vi "OP300ZP_CONTI_HYDRAU.vi"(6 "last?":bool, 7 "OUI/NON":bool, 8 "errin":errorcluster caption="entrée d'erreur (pas d'erreur)", 11 "cluster d'entrée":T1) -> (0 "errout":errorcluster caption="sortie d'erreur")   [LabVIEW 2020]
uses:
  <userlib>/Alex.vi/FGV.ctl
  VG_HYDRAU.vi
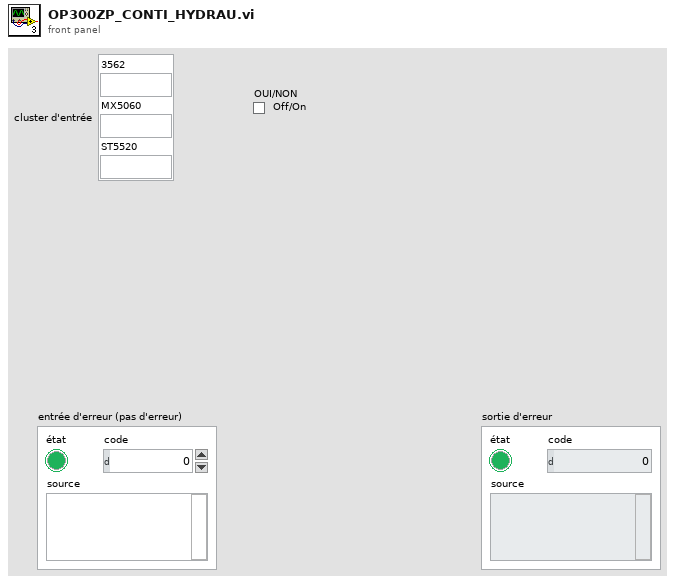
[diagram p1: front panel]
types:
  T1 = cluster{"3562":string, "MX5060":string, "ST5520":string}
  T2 = typedef "FGV.ctl" = enum16{"GET", "SET", "RAZ"}
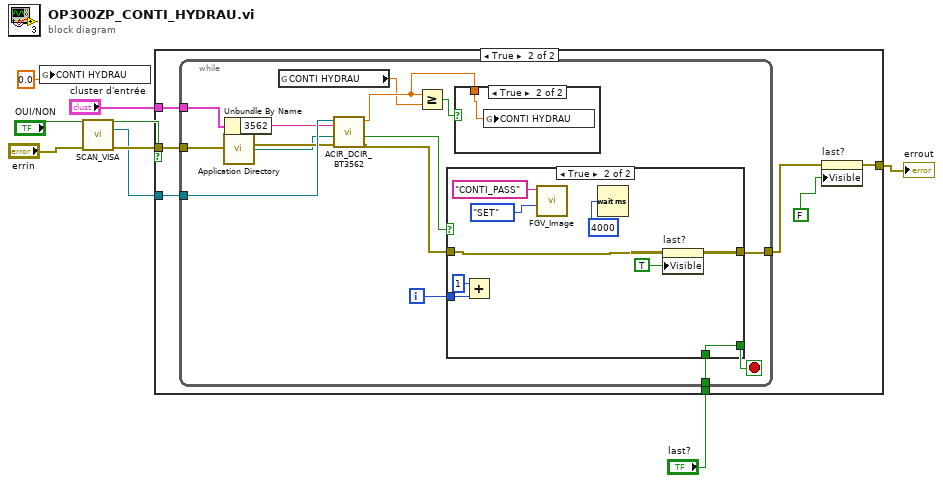
[diagram p0: block diagram]
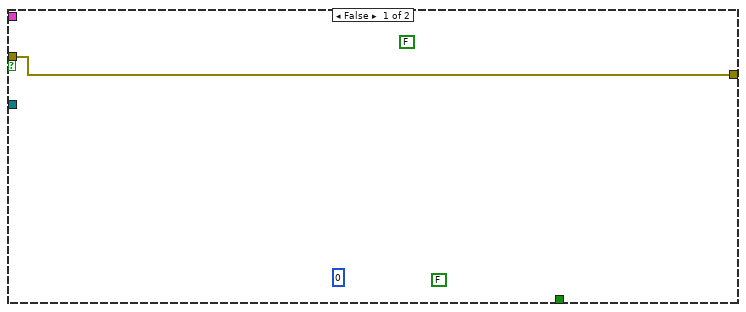
[diagram p2: hidden frame]
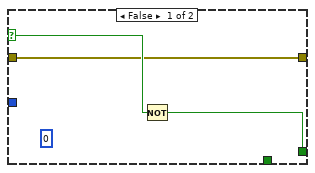
[diagram p3: hidden frame]
diagram:
  n1 = global write "VG_HYDRAU.vi" "CONTI HYDRAU"(0.0 ("R")) -> ()
  n2 = call "SCAN_VISA.vi"("errin"="errin") -> ("sortie d'erreur"=w8:errorcluster, "Refnum VISA en sortie"=w4:refnum<visa-resource-name>)  [unwired: 9 in]
  n3 = case shown="True" "OUI/NON" {
    tunnel: w4 -> [_ w16]
    tunnel: w8 -> [w9 w15]
    tunnel: [w9 w12] -> w7
    tunnel: "cluster d'entrée" -> [_ w14]
    tunnel: "last?" -> [_ w11]
    frame False {
      (unwired) 0
      (unwired) FALSE
      (unwired) FALSE ("OUI/NON")
    }
    frame True {
      n4 = while {
        tunnel: w16 -> [w30]
        tunnel: w15 -> [w29]
        tunnel: [w26] -> w10
        tunnel: w14 -> [w18]
        tunnel: w11 -> [w17]
        i -> [w25]
        stop <- w22 stop-if-true
        n5 = call <vilib>:"Application Directory.vi"() -> ("Application Directory"=w28:path)
        n6 = Unbundle By Name(w18) -> ("3562"=w20:string)
        n7 = global read "VG_HYDRAU.vi" "CONTI HYDRAU"() -> (w19:dbl)
        n8 = call <userlib>:"ACIR_DCIR_BT3562.vi"("errin"=w29, "chemin de base"=w28, "section"=w20, "VISAin"=w30) -> ("errout"=w21:errorcluster, "OK?"=w27:bool, "R"=w23:dbl)  [unwired: 2 in, 3 out]
        n9 = Greater Or Equal?(x=w23, y=w19) -> (x >= y?=w24:bool)
        n10 = case shown="True" w27 {
          selector: w27 -> [w33 _]
          tunnel: w21 -> [w31 w35]
          tunnel: [w31 w37] -> w26
          tunnel: [w32 w34] -> w22
          tunnel: w25 -> [_ w40]
          tunnel: w17 -> [_ w34]
          frame False {
            (unwired) 0
            n11 = Not(x=w33) -> (.not. x?=w32:bool)
          }
          frame True {
            n12 = Add(x=1, y=w40) -> ()  [unwired: 1 out]
            n13 = call <userlib>:"FGV_Image.vi"("Énum"=FGV."SET", "IN"="CONTI_PASS") -> ()  [unwired: 9 in, 1 out]
            n14 = Wait (ms)(milliseconds to wait=u32 4000 ("attente (ms)")) -> ()  [unwired: 1 out]
            n15 = property on="last?" class="Bool"(error in=w35, "Visible"=TRUE) -> (error out=w37:errorcluster)  [unwired: 1 in, 1 out]
          }
        }
        n16 = case shown="True" w24 {
          tunnel: w23 -> [_ w43]
          frame False {
          }
          frame True {
            n17 = global write "VG_HYDRAU.vi" "CONTI HYDRAU"(w43) -> ()
          }
        }
      }
      n18 = property on="last?" class="Bool"(error in=w10, "Visible"=FALSE) -> (error out=w12:errorcluster)  [unwired: 1 in, 1 out]
    }
  }
  "errout" <- w7
